vi "FastHoppingScan.vi"() -> ()   [LabVIEW 2014]
uses:
  <vilib>/userdefined/High Color/nirio_resource_hc.ctl
  <vilib>/Instr/_visa.llb/VISA Configure Serial Port (Instr).vi
  <vilib>/FPGAPlugInAG/PCIe-7851R/niLvFpga_Open_PCIe-7851R.vi
  <vilib>/rvi/interface/common/dynamic/niFpgaDynamicAddResources.vi
  <vilib>/Utility/error.llb/Error Cluster From Error Code.vi
  <vilib>/rvi/errors/niLvFpgaAdjustHostInterfaceError.vi
  <vilib>/FPGAPlugInAG/Dynamic/niLvFpga_Run_Dynamic.vi
  <vilib>/FPGAPlugInAG/Dynamic/niLvFpga_Close_Dynamic.vi
  <vilib>/Analysis/Matrix/Numeric/Conversions/Array To Matrix - RA2.vi
  <vilib>/rvi/interface/nirviOpenFPGA/nirviOpenFPGA.xnode
  FastHoppingModel_FPGATarget_StepApproach_dPgqUSt0PIw.lvbitx
  <vilib>/rvi/interface/nirviReadWriteControl/nirviReadWriteControl.xnode
  <vilib>/rvi/interface/nirviMethod/nirviMethod.xnode
  <vilib>/rvi/interface/nirviCloseFPGA/nirviCloseFPGA.xnode
  NiFpgaLv.dll
  <vilib>/rvi/interface/Simulation/niFpgaSimulationCallBeginRW.vi
  <vilib>/Analysis/Matrix/NI_Matrix.lvlib
  <vilib>/FPGAPlugInAG/Dynamic/niLvFpga_ReadFifo_Dynamic.vi
  <vilib>/rvi/errors/niLvFpgaMergeErrorWithErrorCode.vi
  <vilib>/FPGAPlugInAG/Dynamic/niLvFpga_StopFifo_Dynamic.vi
panel:
  out "Waveform Chart":i16(graph)
  out "ZPos um":dbl
  out "ZPosDia":dbl(graph)
  in  "StepAdjustIndex":i32
  in  "NumToRefresh":u32
  out "DeltaTime ms":u32
  out "ERRIn?":string
  out "XPrePosNum":i32
  out "YPrePosNum":i32
  out "ERROut?":string
  in  "Stop":bool
  in  "Offset":i16
  in  "AppRate us":u32
  in  "Decline %":sgl format="%#_13g"
  in  "PIZ":T1
  in  "YStepLen um":dbl format="%#_13g"
  in  "XStepLen um":dbl format="%#_13g"
  out "YPos um":dbl
  out "XPos um":dbl
  in  "Y Num":i32
  in  "X Num":i32
  in  "YInit um":dbl format="%#_13g"
  in  "XInit um":dbl format="%#_13g"
  in  "RoughXYZ":refnum<visa-resource-name>
  # "3D plot method will cause the labview shut down on this computer!!"
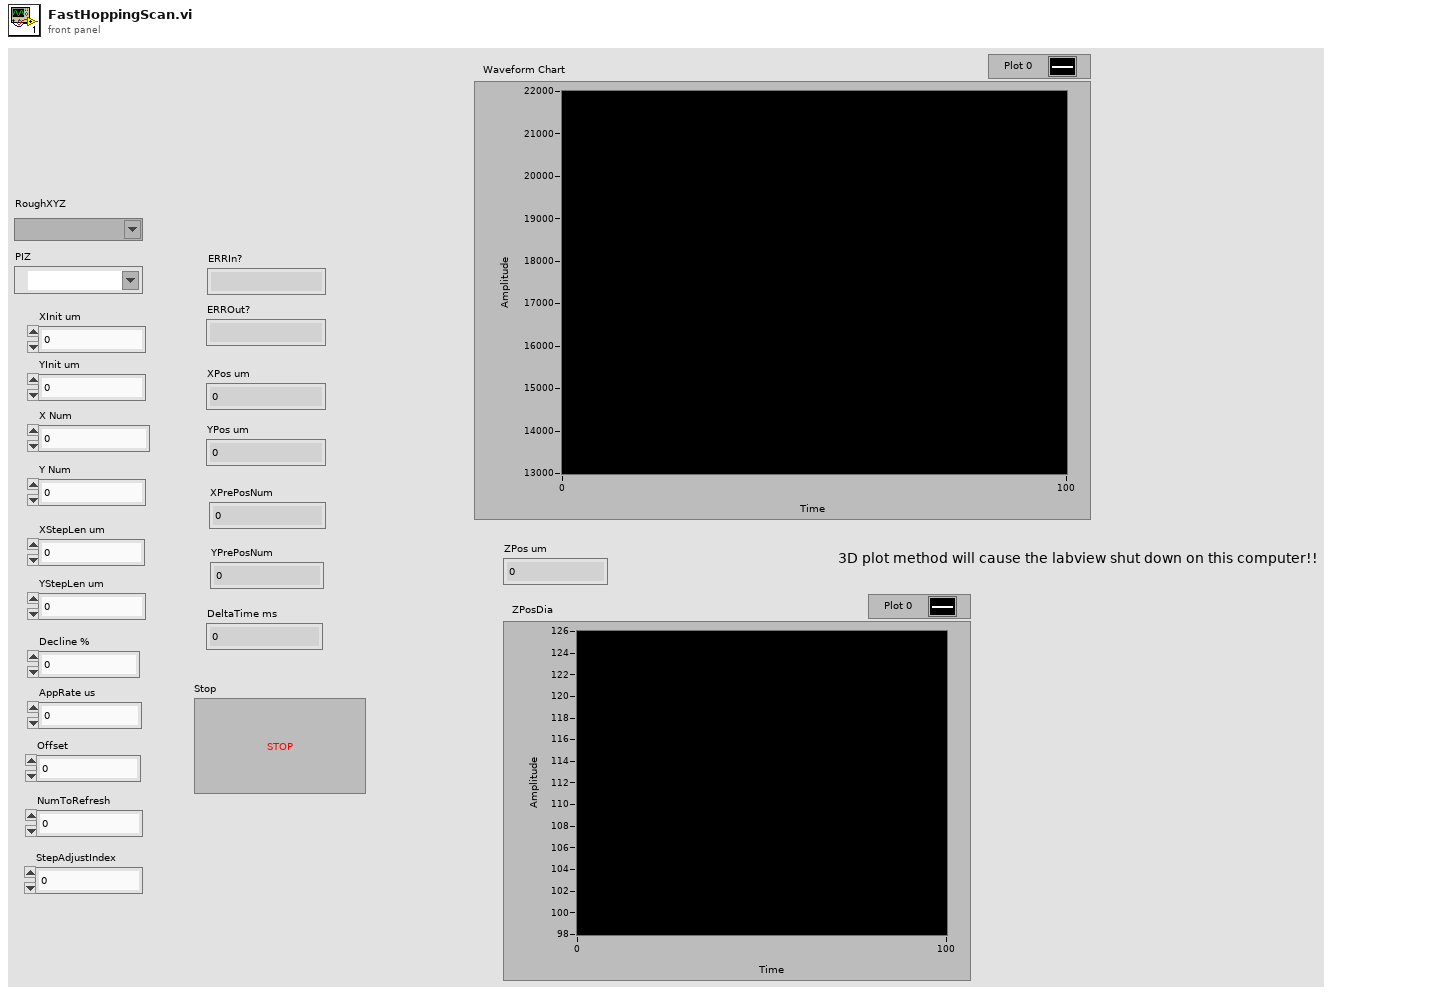
[diagram p1: front panel]
types:
  T1 = typedef "nirio_resource_hc.ctl" = tag
  T2 = typedef "NI_Matrix.lvlib/RealMatrix.ctl" = dbl[][]
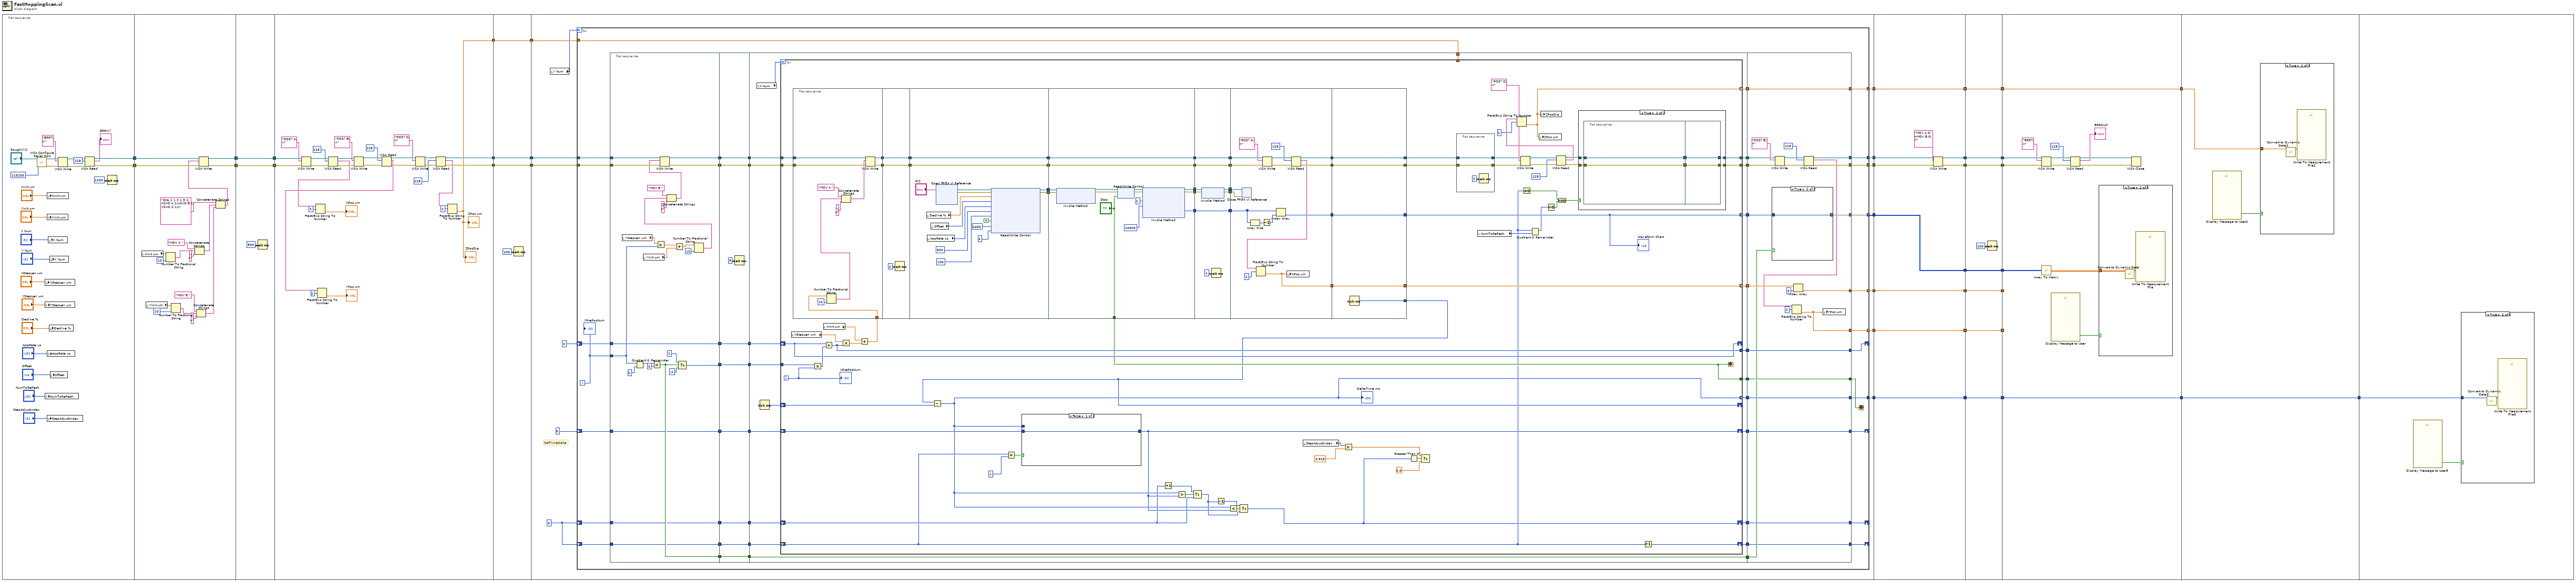
[diagram p0: block diagram]
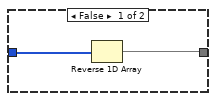
[diagram p4: hidden frame]
diagram:
  n1 = flat-sequence {
    tunnel: [w51] -> w36
    tunnel: [w50] -> w35
    tunnel: w36 -> [w77]
    tunnel: w35 -> [w76]
    tunnel: [w61] -> w34
    tunnel: [w60] -> w33
    tunnel: w34 -> [w80]
    tunnel: w33 -> [w79]
    tunnel: [w80] -> w32
    tunnel: [w79] -> w31
    tunnel: w32 -> [w109]
    tunnel: w31 -> [w108]
    tunnel: [w85] -> w30
    tunnel: [w84] -> w29
    tunnel: [w81] -> w6
    tunnel: w30 -> [w112]
    tunnel: w29 -> [w111]
    tunnel: [w112] -> w28
    tunnel: [w111] -> w27
    tunnel: [w110] -> w7
    tunnel: w6 -> [w110]
    tunnel: w28 -> [w126]
    tunnel: w27 -> [w125]
    tunnel: [w123] -> w26
    tunnel: [w122] -> w25
    tunnel: [w121] -> w24
    tunnel: [w120] -> w23
    tunnel: [w119] -> w22
    tunnel: [w116] -> w11
    tunnel: w7 -> [w115]
    tunnel: [w114] -> w5
    tunnel: w26 -> [w431]
    tunnel: w25 -> [w430]
    tunnel: w24 -> [w432]
    tunnel: w23 -> [w433]
    tunnel: w22 -> [w434]
    tunnel: [w434] -> w20
    tunnel: [w433] -> w18
    tunnel: [w432] -> w16
    tunnel: [w429] -> w15
    tunnel: [w428] -> w12
    tunnel: w11 -> [w426]
    tunnel: [w426] -> w8
    tunnel: w5 -> [w425]
    tunnel: [w425] -> w3
    tunnel: [w442] -> w21
    tunnel: w20 -> [w442]
    tunnel: [w441] -> w19
    tunnel: w18 -> [w441]
    tunnel: [w440] -> w17
    tunnel: w16 -> [w440]
    tunnel: w15 -> [w439]
    tunnel: [w439] -> w14
    tunnel: [w438] -> w13
    tunnel: w12 -> [w438]
    tunnel: [w436] -> w9
    tunnel: w8 -> [w436]
    tunnel: [w435] -> w4
    tunnel: w3 -> [w435]
    tunnel: w21 -> [_]
    tunnel: w19 -> [_]
    tunnel: w17 -> [w449]
    tunnel: w14 -> [w452]
    tunnel: w13 -> [w451]
    tunnel: [w444] -> w10
    tunnel: w9 -> [w444]
    tunnel: w4 -> [w443]
    tunnel: [w443] -> w2
    tunnel: w10 -> [w460]
    tunnel: w2 -> [w459]
    tunnel: [w459] -> w1
    tunnel: w1 -> [w464]
    frame #0 {
      n2 = call-poly "VISA Configure Serial Port"("VISA resource name"="RoughXYZ", "baud rate (9600)"=u32 115200) -> ("VISA resource name out"=w57:refnum<visa-resource-name>, "error out"=w56:errorcluster)  [unwired: 12 in]
      n3 = local write "XStepLen um"("XStepLen um") -> ()
      n4 = local write "YStepLen um"("YStepLen um") -> ()
      n5 = local write "NumToRefresh"("NumToRefresh") -> ()
      n6 = local write "XInit um"("XInit um") -> ()
      n7 = local write "YInit um"("YInit um") -> ()
      n8 = local write "StepAdjustIndex"("StepAdjustIndex") -> ()
      n9 = local write "AppRate us"("AppRate us") -> ()
      n10 = local write "X Num"("X Num") -> ()
      n11 = local write "Decline %"("Decline %") -> ()
      n12 = local write "Y Num"("Y Num") -> ()
      n13 = local write "Offset"("Offset") -> ()
      n14 = VISA Write(VISA resource name=w57, write buffer="ERR?\n", error in (no error)=w56) -> (VISA resource name out=w54:refnum<visa-resource-name>, error out=w53:errorcluster)  [unwired: 1 out]
      n15 = VISA Read(VISA resource name=w54, byte count=u32 128, error in (no error)=w53) -> (VISA resource name out=w51:refnum<visa-resource-name>, read buffer=→"ERRIn?":string, error out=w50:errorcluster)  [unwired: 1 out]
      n16 = Wait (ms)(milliseconds to wait=u32 1200) -> ()  [unwired: 1 out]
    }
    frame #1 {
      n17 = local read "XInit um"() -> (w73:dbl)
      n18 = local read "YInit um"() -> (w69:dbl)
      n19 = Number To Fractional String(number=w73, precision (6)=i16 10) -> (F-format string=w71:string)  [unwired: 2 in]
      n20 = Number To Fractional String(number=w69, precision (6)=i16 10) -> (F-format string=w67:string)  [unwired: 2 in]
      n21 = Concatenate Strings("MOV A " ("string"), w71, "\n" ("string")) -> (w64:string)
      n22 = Concatenate Strings("MOV B " ("string"), w67, "\n" ("string")) -> (w63:string)
      n23 = Concatenate Strings("ONL 1 1 2 1 3 1\nSVO A 1\nSVO B 1\nSVO C 1\n" ("write buffer"), w64, w63) -> (w62:string)
      n24 = VISA Write(VISA resource name=w77, write buffer=w62, error in (no error)=w76) -> (VISA resource name out=w61:refnum<visa-resource-name>, error out=w60:errorcluster)  [unwired: 1 out]
    }
    frame #2 {
      n25 = Wait (ms)(milliseconds to wait=u32 500) -> ()  [unwired: 1 out]
    }
    frame #3 {
      n26 = VISA Write(VISA resource name=w109, write buffer="POS? A\n", error in (no error)=w108) -> (VISA resource name out=w106:refnum<visa-resource-name>, error out=w105:errorcluster)  [unwired: 1 out]
      n27 = VISA Read(VISA resource name=w106, byte count=u32 128, error in (no error)=w105) -> (VISA resource name out=w102:refnum<visa-resource-name>, read buffer=w97:string, error out=w101:errorcluster)  [unwired: 1 out]
      n28 = Fract/Exp String To Number(string=w97, offset=2) -> (number=→"XPos um":dbl)  [unwired: 2 in, 1 out]
      n29 = VISA Write(VISA resource name=w102, write buffer="POS? B\n", error in (no error)=w101) -> (VISA resource name out=w100:refnum<visa-resource-name>, error out=w99:errorcluster)  [unwired: 1 out]
      n30 = VISA Read(VISA resource name=w100, byte count=u32 128, error in (no error)=w99) -> (VISA resource name out=w91:refnum<visa-resource-name>, read buffer=w94:string, error out=w90:errorcluster)  [unwired: 1 out]
      n31 = Fract/Exp String To Number(string=w94, offset=2) -> (number=→"YPos um":dbl)  [unwired: 2 in, 1 out]
      n32 = VISA Write(VISA resource name=w91, write buffer="POS? C\n", error in (no error)=w90) -> (VISA resource name out=w89:refnum<visa-resource-name>, error out=w88:errorcluster)  [unwired: 1 out]
      n33 = VISA Read(VISA resource name=w89, byte count=u32 128, error in (no error)=w88) -> (VISA resource name out=w85:refnum<visa-resource-name>, read buffer=w82:string, error out=w84:errorcluster)  [unwired: 1 out]
      n34 = Fract/Exp String To Number(string=w82, offset=2) -> (number=w81:dbl)  [unwired: 2 in, 1 out]
      "ZPosDia" <- w81
      "ZPos um" <- w81
    }
    frame #4 {
      n35 = Wait (ms)(milliseconds to wait=u32 100) -> ()  [unwired: 1 out]
    }
    frame #5 {
      w117 = i64 0
      # "RefTimeDelta"
      n36 = local read "Y Num"() -> (w127:i32)
      n37 = for {
        N: w127 -> [_]
        tunnel: w126 -> [w175]
        tunnel: w125 -> [w174]
        shift-right: [w157] -> _
        shift-left: 0 -> [w159]
        tunnel: [w156] -> w123
        tunnel: [w155] -> w122
        tunnel: [w154] -> w121 mode=indexing
        tunnel: [w153] -> w120 mode=indexing
        tunnel: [w152] -> w119 mode=indexing
        shift-right: [w145] -> _
        shift-left: w117 -> [w143]
        shift-right: [w140] -> _
        shift-left: 0 -> [w138]
        shift-right: [w134] -> _
        shift-left: w117 -> [w133]
        tunnel: [w131] -> w116 mode=concatenating
        tunnel: w115 -> [w130]
        tunnel: [w129] -> w114 mode=concatenating
        i -> [w173]
        stop <- w163 stop-if-true
        n38 = flat-sequence {
          tunnel: w175 -> [w200]
          tunnel: w174 -> [w199]
          tunnel: w173 -> [w190]
          tunnel: [w192] -> w172
          tunnel: [w191] -> w171
          tunnel: [w186] -> w170
          tunnel: w159 -> [w185]
          tunnel: [w185] -> w167
          tunnel: [w179] -> w149
          tunnel: [w178] -> w146
          tunnel: w143 -> [w178]
          tunnel: [w177] -> w141
          tunnel: w138 -> [w177]
          tunnel: [w176] -> w136
          tunnel: w133 -> [w176]
          tunnel: w172 -> [w208]
          tunnel: w171 -> [w207]
          tunnel: w170 -> [w205]
          tunnel: [w208] -> w169
          tunnel: [w207] -> w168
          tunnel: w167 -> [w206]
          tunnel: [w206] -> w166
          tunnel: [w205] -> w165
          tunnel: [w204] -> w150
          tunnel: w149 -> [w204]
          tunnel: [w203] -> w147
          tunnel: w146 -> [w203]
          tunnel: [w202] -> w142
          tunnel: w141 -> [w202]
          tunnel: [w201] -> w137
          tunnel: w136 -> [w201]
          tunnel: w169 -> [w229]
          tunnel: w168 -> [w228]
          tunnel: w166 -> [w230]
          tunnel: w165 -> [w227]
          tunnel: [w226] -> w164
          tunnel: [w225] -> w162
          tunnel: [w224] -> w161
          tunnel: [w223] -> w160
          tunnel: [w222] -> w158
          tunnel: [w221] -> w151
          tunnel: w150 -> [w219]
          tunnel: [w219] -> w148
          tunnel: w147 -> [w218]
          tunnel: [w217] -> w144
          tunnel: w142 -> [w216]
          tunnel: [w215] -> w139
          tunnel: w137 -> [w213]
          tunnel: [w214] -> w135
          tunnel: [w212] -> w132
          tunnel: w130 -> [w211]
          tunnel: [w210] -> w128
          tunnel: w164 -> [w421]
          tunnel: [w421] -> w163
          tunnel: w162 -> [w404]
          tunnel: w161 -> [w416]
          tunnel: w160 -> [w415]
          tunnel: w158 -> [w414]
          tunnel: [w414] -> w157
          tunnel: [w413] -> w156
          tunnel: [w412] -> w155
          tunnel: [w403] -> w154
          tunnel: [w409] -> w153
          tunnel: [w406] -> w152
          tunnel: w151 -> [w408]
          tunnel: w148 -> [w405]
          tunnel: [w402] -> w145
          tunnel: w144 -> [w402]
          tunnel: [w401] -> w140
          tunnel: w139 -> [w401]
          tunnel: w135 -> [w400]
          tunnel: [w400] -> w134
          tunnel: w132 -> [w399]
          tunnel: [w399] -> w131
          tunnel: [w398] -> w129
          tunnel: w128 -> [w398]
          frame #0 {
            n39 = local read "YStepLen um"() -> (w198:dbl)
            n40 = Quotient & Remainder(x=w190, y=2) -> (x-y*floor(x/y)=w188:i32)  [unwired: 1 out]
            n41 = local read "YInit um"() -> (w181:dbl)
            n42 = Equal?(x=w188, y=0) -> (x = y?=w179:bool)
            n43 = Multiply(x=w198, y=w190) -> (x*y=w182:dbl)
            n44 = Add(x=w182, y=w181) -> (x+y=w180:dbl)
            n45 = Select(t=1 ("y"), s=w179, f=-1 ("y")) -> (s? t:f=w186:i32)
            n46 = Number To Fractional String(number=w180, precision (6)=i16 10) -> (F-format string=w194:string)  [unwired: 2 in]
            n47 = Concatenate Strings("MOV B " ("string"), w194, "\n" ("string")) -> (w193:string)
            n48 = VISA Write(VISA resource name=w200, write buffer=w193, error in (no error)=w199) -> (VISA resource name out=w192:refnum<visa-resource-name>, error out=w191:errorcluster)  [unwired: 1 out]
          }
          frame #1 {
            n49 = Wait (ms)(milliseconds to wait=u32 5) -> ()  [unwired: 1 out]
          }
          frame #2 {
            n50 = local read "X Num"() -> (w231:i32)
            n51 = Tick Count (ms)() -> (millisecond timer value=w220:u32)
            n52 = for {
              N: w231 -> [_]
              tunnel: w229 -> [w308]
              tunnel: w228 -> [w307]
              tunnel: w227 -> [w297]
              tunnel: [w300] -> w226
              tunnel: [w234] -> w225 mode=indexing
              tunnel: [w272] -> w224
              tunnel: [w271] -> w223
              shift-right: [w294] -> _
              shift-left: w230 -> [w294]
              tunnel: [w293] -> w222
              tunnel: [w289] -> w221 mode=indexing
              shift-right: [w273] -> _
              shift-left: w220 -> [w288]
              shift-right: [w266] -> w215
              shift-left: w216 -> [w270]
              shift-right: [w251] -> w217
              shift-left: w218 -> [w263]
              shift-right: [w259] -> w214
              shift-left: w213 -> [w256]
              tunnel: [w238] -> w212 mode=indexing
              tunnel: w211 -> [_]
              tunnel: [w235] -> w210 mode=indexing
              i -> [w261]
              stop <- w300 stop-if-true
              n53 = local read "XStepLen um"() -> (w295:dbl)
              n54 = flat-sequence {
                tunnel: w308 -> [w335]
                tunnel: w307 -> [w334]
                tunnel: [w332] -> w306
                tunnel: [w331] -> w305
                tunnel: w292 -> [w326]
                tunnel: w306 -> [w337]
                tunnel: w305 -> [w336]
                tunnel: [w337] -> w304
                tunnel: [w336] -> w303
                tunnel: w304 -> [w343]
                tunnel: w303 -> [w342]
                tunnel: [w345] -> w302
                tunnel: [w344] -> w301
                tunnel: [w343] -> w299
                tunnel: [w342] -> w298
                tunnel: w302 -> [w357]
                tunnel: w301 -> [w356]
                tunnel: ["Stop"] -> w300
                tunnel: w299 -> [w362]
                tunnel: [w362] -> w287
                tunnel: [w361] -> w285
                tunnel: w298 -> [w361]
                tunnel: [w360] -> w283
                tunnel: [w359] -> w281
                tunnel: [w358] -> w279
                tunnel: w287 -> [w375]
                tunnel: [w375] -> w286
                tunnel: w285 -> [w374]
                tunnel: [w374] -> w284
                tunnel: w283 -> [w371]
                tunnel: [w369] -> w282
                tunnel: w281 -> [w370]
                tunnel: [w368] -> w280
                tunnel: w279 -> [w373]
                tunnel: [w373] -> w278
                tunnel: w286 -> [w392]
                tunnel: w284 -> [w391]
                tunnel: w282 -> [w384]
                tunnel: w280 -> [w383]
                tunnel: w278 -> [w382]
                tunnel: [w386] -> w277
                tunnel: [w385] -> w276
                tunnel: [w381] -> w275
                tunnel: [w376] -> w274
                tunnel: [w395] -> w289
                tunnel: [w396] -> w234
                tunnel: [w397] -> w233
                tunnel: w277 -> [w397]
                tunnel: w276 -> [w393]
                tunnel: w275 -> [w396]
                tunnel: w274 -> [w395]
                tunnel: [w394] -> w273
                tunnel: [w393] -> w232
                frame #0 {
                  n55 = Number To Fractional String(number=w326, precision (6)=i16 10) -> (F-format string=w327:string)  [unwired: 2 in]
                  n56 = Concatenate Strings("MOV A " ("string"), w327, "\n" ("string")) -> (w328:string)
                  n57 = VISA Write(VISA resource name=w335, write buffer=w328, error in (no error)=w334) -> (VISA resource name out=w332:refnum<visa-resource-name>, error out=w331:errorcluster)  [unwired: 1 out]
                }
                frame #1 {
                  n58 = Wait (ms)(milliseconds to wait=u32 2) -> ()  [unwired: 1 out]
                }
                frame #2 {
                  n59 = local read "Decline %"() -> (w350:sgl)
                  n60 = local read "AppRate us"() -> (w348:u32)
                  n61 = local read "Offset"() -> (w349:i16)
                  n62 = xnode ("Open FPGA VI Reference")("resource name"="PIZ") -> ("FPGA VI Reference Out"=w352:refnum<k20>, "error out"=w351:errorcluster)  [unwired: 1 in]
                  n63 = xnode "Read/Write Control"("FPGA VI Reference In"=w352, "error in"=w351, "Percentage %"=w350, "Offset"=w349, "AppRate us"=w348, "BaseTime us"=u32 500, "CurrSampleNum"=u32 100, "SeveralSampleMeasure?"=TRUE, "WithdrawStep"=i16 1000, "MeasureCount"=i16 4) -> ("FPGA VI Reference Out"=w345:refnum<k20>, "error out"=w344:errorcluster)
                }
                frame #3 {
                  n64 = xnode "Invoke Method"("FPGA VI Reference In"=w357, "error in"=w356) -> ("FPGA VI Reference Out"=w355:refnum<k20>, "error out"=w354:errorcluster)  [unwired: 1 in]
                  n65 = xnode "Read/Write Control"("FPGA VI Reference In"=w355, "error in"=w354, "stop"="Stop") -> ("FPGA VI Reference Out"=w367:refnum<k20>, "error out"=w366:errorcluster)
                  n66 = xnode "Invoke Method"("FPGA VI Reference In"=w367, "error in"=w366, "Number of Elements"=u32 1, "Timeout (ms)"=10000) -> ("FPGA VI Reference Out"=w360:refnum<k20>, "error out"=w359:errorcluster, "Data"=w358:i16[])  [unwired: 1 out]
                }
                frame #4 {
                  n67 = xnode "Invoke Method"("FPGA VI Reference In"=w371, "error in"=w370) -> ("FPGA VI Reference Out"=w369:refnum<k20>, "error out"=w368:errorcluster)
                  n68 = Wait (ms)(milliseconds to wait=u32 1) -> ()  [unwired: 1 out]
                }
                frame #5 {
                  n69 = xnode "Close FPGA VI Reference"("FPGA VI Reference In"=w384, "error in"=w383) -> ()  [unwired: 1 out]
                  n70 = Array Size(array=w382) -> (size(s)=w380:i32)
                  n71 = Decrement(x=w380) -> (x-1=w379:i32)
                  n72 = VISA Write(VISA resource name=w392, write buffer="POS? A\n", error in (no error)=w391) -> (VISA resource name out=w389:refnum<visa-resource-name>, error out=w388:errorcluster)  [unwired: 1 out]
                  n73 = Index Array(array=w382, index=w379) -> (element=w381:i16)
                  n74 = VISA Read(VISA resource name=w389, byte count=u32 128, error in (no error)=w388) -> (VISA resource name out=w386:refnum<visa-resource-name>, read buffer=w378:string, error out=w385:errorcluster)  [unwired: 1 out]
                  n75 = Fract/Exp String To Number(string=w378, offset=2) -> (number=w376:dbl)  [unwired: 2 in, 1 out]
                  n76 = local write "XPos um"(w376) -> ()
                }
                frame #6 {
                  n77 = Tick Count (ms)() -> (millisecond timer value=w394:u32)
                }
              }
              n78 = Multiply(x=w297, y=w261) -> (x*y=w296:i32)
              n79 = local read "XInit um"() -> (w290:dbl)
              n80 = Add(x=w294, y=w296) -> (x+y=w293:i32)
              n81 = Multiply(x=w295, y=w293) -> (x*y=w291:dbl)
              n82 = Add(x=w290, y=w291) -> (x+y=w292:dbl)
              n83 = Subtract(x=w273, y=w288) -> (x-y=w235:u32)
              "DeltaTime ms" <- w235
              n84 = Equal?(x=w256, y=1) -> (x = y?=w262:bool)
              n85 = case shown="False" w262 {
                tunnel: w235 -> [_ w313]
                tunnel: w270 -> [w312 _]
                tunnel: [w312 w313] -> w266
                frame False {
                }
                frame True {
                }
              }
              n86 = Increment(x=w263) -> (x+1=w268:i64)
              n87 = Greater?(x=w235, y=w266) -> (0:w269:bool)
              n88 = Select(t=w268, s=w269, f=w263) -> (s? t:f=w264:i64)
              n89 = Decrement(x=w264) -> (x-1=w265:i64)
              n90 = Less?(x=w235, y=w266) -> (x < y?=w267:bool)
              n91 = Select(t=w265, s=w267, f=w264) -> (s? t:f=w251:i64)
              n92 = local read "StepAdjustIndex"() -> (w249:i32)
              n93 = Multiply(x=w249, y=0.915) -> (x*y=w248:dbl)
              n94 = Greater Than 0?(x=w251) -> (x > 0?=w252:bool)
              n95 = Select(t=w248, s=w252, f=0.0) -> ()  [unwired: 1 out]
              n96 = flat-sequence {
                tunnel: w233 -> [w311]
                tunnel: w232 -> [w310]
                tunnel: [w311] -> w237
                tunnel: [w310] -> w236
                frame #0 {
                  n97 = Wait (ms)(milliseconds to wait=u32 2) -> ()  [unwired: 1 out]
                }
              }
              n98 = local read "NumToRefresh"() -> (w258:u32)
              n99 = VISA Write(VISA resource name=w237, write buffer="POS? C\n", error in (no error)=w236) -> (VISA resource name out=w244:refnum<visa-resource-name>, error out=w243:errorcluster)  [unwired: 1 out]
              n100 = Not Equal To 0?(x=w256) -> (x != 0?=w255:bool)
              n101 = Quotient & Remainder(x=w256, y=w258) -> (x-y*floor(x/y)=w254:i64)  [unwired: 1 out]
              n102 = Equal To 0?(x=w254) -> (x = 0?=w253:bool)
              n103 = VISA Read(VISA resource name=w244, byte count=u32 128, error in (no error)=w243) -> (VISA resource name out=w246:refnum<visa-resource-name>, read buffer=w239:string, error out=w245:errorcluster)  [unwired: 1 out]
              n104 = Fract/Exp String To Number(string=w239, offset=2) -> (number=w238:dbl)  [unwired: 2 in, 1 out]
              n105 = local write "ZPos um"(w238) -> ()
              n106 = local write "ZPosDia"(w238) -> ()
              n107 = And(x=w255, y=w253) -> (x .and. y?=w257:bool)
              n108 = case shown="True" w257 {
                tunnel: w246 -> [w315 w321]
                tunnel: w245 -> [w314 w320]
                tunnel: [w315 w319] -> w272
                tunnel: [w314 w317] -> w271
                frame False {
                }
                frame True {
                  n109 = flat-sequence {
                    tunnel: w321 -> [w323]
                    tunnel: w320 -> [w322]
                    tunnel: [w323] -> w318
                    tunnel: [w322] -> w316
                    tunnel: [w325] -> w319
                    tunnel: w318 -> [w325]
                    tunnel: [w324] -> w317
                    tunnel: w316 -> [w324]
                    frame #0 {
                    }
                    frame #1 {
                    }
                  }
                }
              }
              n110 = Increment(x=w256) -> (x+1=w259:i64)
              "XPrePosNum" <- w261
              "Waveform Chart" <- w234
            }
          }
          frame #3 {
            n111 = case shown="True" w405 {
              tunnel: w404 -> [w423 w424]
              tunnel: [w422 w424] -> w403
              frame False {
                n112 = Reverse 1D Array(array=w423) -> (reversed array=w422:i16[])
              }
              frame True {
              }
            }
            n113 = VISA Write(VISA resource name=w416, write buffer="POS? B\n", error in (no error)=w415) -> (VISA resource name out=w419:refnum<visa-resource-name>, error out=w418:errorcluster)  [unwired: 1 out]
            n114 = Index Array(array=w408, index=0) -> (element=w406:dbl)
            n115 = VISA Read(VISA resource name=w419, byte count=u32 128, error in (no error)=w418) -> (VISA resource name out=w413:refnum<visa-resource-name>, read buffer=w410:string, error out=w412:errorcluster)  [unwired: 1 out]
            n116 = Fract/Exp String To Number(string=w410, offset=2) -> (number=w409:dbl)  [unwired: 2 in, 1 out]
            n117 = local write "YPos um"(w409) -> ()
          }
        }
        "YPrePosNum" <- w173
      }
    }
    frame #6 {
      n118 = VISA Write(VISA resource name=w431, write buffer="MOV A 0\nMOV B 0\n", error in (no error)=w430) -> (VISA resource name out=w429:refnum<visa-resource-name>, error out=w428:errorcluster)  [unwired: 1 out]
    }
    frame #7 {
      n119 = Wait (ms)(milliseconds to wait=u32 200) -> ()  [unwired: 1 out]
    }
    frame #8 {
      n120 = VISA Write(VISA resource name=w452, write buffer="ERR?\n", error in (no error)=w451) -> (VISA resource name out=w455:refnum<visa-resource-name>, error out=w454:errorcluster)  [unwired: 1 out]
      n121 = call-poly <vilib>:"Array To Matrix.vi"("Real 2D Array"=w449) -> ("Real Matrix"=w445:T2)
      n122 = call "Display Message to User"() -> ("OK"=w446:bool)  [unwired: 10 in, 1 out]
      n123 = VISA Read(VISA resource name=w455, byte count=u32 128, error in (no error)=w454) -> (VISA resource name out=w448:refnum<visa-resource-name>, read buffer=→"ERROut?":string, error out=w447:errorcluster)  [unwired: 1 out]
      n124 = case shown="True" w446 {
        tunnel: w445 -> [_ w458]
        frame False {
        }
        frame True {
          n125 = call "Convert to Dynamic Data"("2D Array"=w458) -> ("Dynamic Data Type"=w457:dynamicdata)  [unwired: 3 in]
          n126 = call "Write To Measurement File"("Signals"=w457) -> ()  [unwired: 16 in, 3 out]
        }
      }
      n127 = VISA Close(VISA resource name=w448, error in (no error)=w447) -> ()  [unwired: 1 out]
    }
    frame #9 {
      n128 = call "Display Message to User2"() -> ("OK"=w461:bool)  [unwired: 10 in, 1 out]
      n129 = case shown="True" w461 {
        tunnel: w460 -> [_ w463]
        frame False {
        }
        frame True {
          n130 = call "Convert to Dynamic Data2"("Array"=w463) -> ("Dynamic Data Type"=w462:dynamicdata)  [unwired: 3 in]
          n131 = call "Write To Measurement File2"("Signals"=w462) -> ()  [unwired: 16 in, 3 out]
        }
      }
    }
    frame #10 {
      n132 = call "Display Message to User3"() -> ("OK"=w465:bool)  [unwired: 10 in, 1 out]
      n133 = case shown="True" w465 {
        tunnel: w464 -> [_ w467]
        frame False {
        }
        frame True {
          n134 = call "Convert to Dynamic Data3"("Array"=w467) -> ("Dynamic Data Type"=w466:dynamicdata)  [unwired: 3 in]
          n135 = call "Write To Measurement File3"("Signals"=w466) -> ()  [unwired: 16 in, 3 out]
        }
      }
    }
  }
